vi "Receive Message.vi"(6 "priority":i32, 10 "Child_2_Class in":refnum<class "Console_Class.lvclass">, 11 "Message in":refnum<class "Message.lvclass">) -> (0 "error out":errorcluster, 2 "Actor out":refnum<class "Actor.lvclass">)   [LabVIEW 2023, in "Console_Actor.lvlib" / "Console_Class.lvclass"]
doc: "This VI should be overriden ONLY if you are creating a proxy actor for remote transmission. If you are, override this VI to transmit the received message to a new destination, maintaining the given priority."
uses:
  Console_Class.lvclass
  <vilib>/ActorFramework/Message/Message.lvclass
  <vilib>/ActorFramework/Actor/Actor.lvclass
  Abstraction_Interface_Class/Abstraction_Interface_Class.lvclass
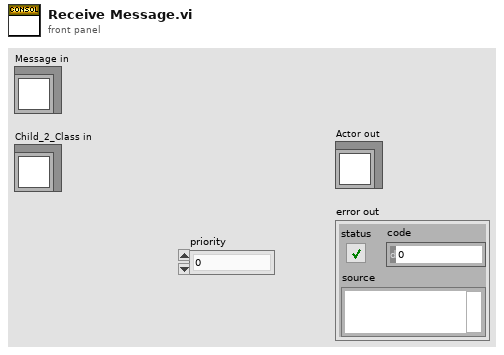
[diagram p1: front panel]
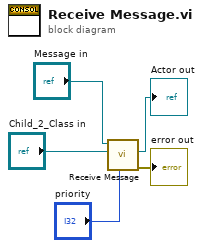
[diagram p0: block diagram]
diagram:
  n1 = call-parent "Receive Message.vi"("priority"="priority", "Actor in"="Child_2_Class in", "Message in"="Message in") -> ("error out"=→"error out":errorcluster, "Actor out"=→"Actor out":refnum<class "Actor.lvclass">)  [unwired: 7 in]
